vi "Button Toggle Solenoid Climb_Cylinder.vi"(11 "Button A":bool) -> (3 "Climb_Cylinder_Value":T1)   [LabVIEW 2020]
uses:
  <vilib>/Rock Robotics/WPI/Solenoid/WPI_SolenoidValue.ctl
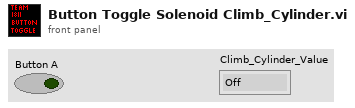
[diagram p1: front panel]
types:
  T1 = typedef "WPI_SolenoidValue.ctl" = enum16{"Off", "On", "Forward", "Reverse"}
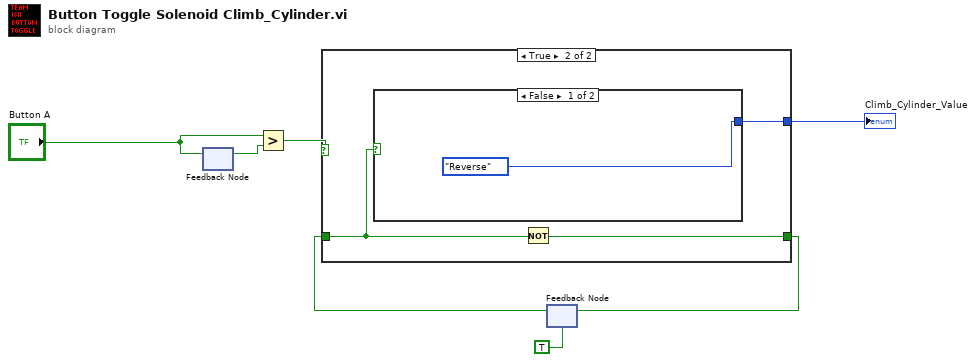
[diagram p0: block diagram]
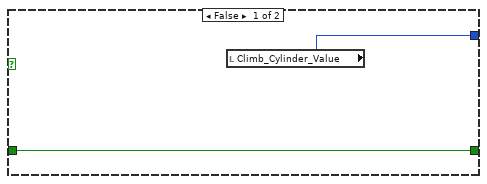
[diagram p2: hidden frame]
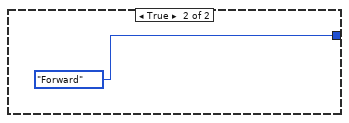
[diagram p3: hidden frame]
diagram:
  n1 = feedback #1() -> (w6:bool)  [unwired: 1 in]
  n2 = feedback-in #1("Button A") -> ()
  n3 = Greater?(x="Button A", y=w6) -> (0:w7:bool)
  n4 = feedback #2(TRUE) -> (w5:bool)
  n5 = case shown="True" w7 {
    tunnel: w5 -> [w9 w11]
    tunnel: [w9 w12] -> w4
    tunnel: [w8 w10] -> w1
    frame False {
      n6 = local read "Climb_Cylinder_Value"() -> (w8:T1)
    }
    frame True {
      n7 = case shown="False" w11 {
        tunnel: [WPI_SolenoidValue."Reverse" ("Climb_Cylinder") WPI_SolenoidValue."Forward" ("Climb_Cylinder")] -> w10
        frame False {
        }
        frame True {
        }
      }
      n8 = Not(x=w11) -> (.not. x?=w12:bool)
    }
  }
  "Climb_Cylinder_Value" <- w1
  n9 = feedback-in #2(w4) -> ()
